vi "rs3_stream_decode3.vi"(8 "error in":errorcluster, 10 "Stream Profile Array":T2(array[cluster])=[{"ID"=1, "Profile"=389917496, "fps"=25, "RS Stream"=3, "RS Format"=0, "index"=1, "width"=1920, "height"=1080, "ppx"=0.0, "ppy"=0.0, "fx"=0.0, "fy"=0.0, "model"=0}, {"ID"=2, "Profile"=389920056, "fps"=25, "RS Stream"=3, "RS Format"=0, "index"=2, "width"=1920, "height"=1080, "ppx"=0.0, "ppy"=0.0, "fx"=0.0, "fy"=0.0, "model"=0}, {"ID"=2, "Profile"=389913400, "fps"=25, "RS Stream"=3, "RS Format"=0, "index"=2, "width"=1920, "height"=1080, "ppx"=946.5989, "ppy"=565.6723, "fx"=1415.005, "fy"=1415.005, "model"=4}, {"ID"=1, "Profile"=389905464, "fps"=25, "RS Stream"=3, "RS Format"=0, "index"=1, "width"=1920, "height"=1080, "ppx"=946.5989, "ppy"=565.6723, "fx"=1415.005, "fy"=1415.005, "model"=4}, {"ID"=1, "Profile"=389918776, "fps"=15, "RS Stream"=3, "RS Format"=0, "index"=1, "width"=1920, "height"=1080, "ppx"=0.0, "ppy"=0.0, "fx"=0.0, "fy"=0.0, "model"=0}, {"ID"=2, "Profile"=389918264, "fps"=15, "RS Stream"=3, "RS Format"=0, "index"=2, "width"=1920, "height"=1080, "ppx"=0.0, "ppy"=0.0, "fx"=0.0, "fy"=0.0, "model"=0}, {"ID"=2, "Profile"=389917240, "fps"=15, "RS Stream"=3, "RS Format"=0, "index"=2, "width"=1920, "height"=1080, "ppx"=946.5989, "ppy"=565.6723, "fx"=1415.005, "fy"=1415.005, "model"=4}, {"ID"=1, "Profile"=389916728, "fps"=15, "RS Stream"=3, "RS Format"=0, "index"=1, "width"=1920, "height"=1080, "ppx"=946.5989, "ppy"=565.6723, "fx"=1415.005, "fy"=1415.005, "model"=4}, {"ID"=1, "Profile"=389901608, "fps"=30, "RS Stream"=3, "RS Format"=0, "index"=0, "width"=1280, "height"=720, "ppx"=631.0659, "ppy"=377.11487, "fx"=943.3367, "fy"=943.3367, "model"=4}, {"ID"=1, "Profile"=389892136, "fps"=30, "RS Stream"=3, "RS Format"=0, "index"=0, "width"=1280, "height"=720, "ppx"=0.0, "ppy"=0.0, "fx"=0.0, "fy"=0.0, "model"=0}, {"ID"=1, "Profile"=389461048, "fps"=30, "RS Stream"=3, "RS Format"=0, "index"=1, "width"=1280, "height"=720, "ppx"=631.0659, "ppy"=377.11487, "fx"=943.3367, "fy"=943.3367, "model"=4}, {"ID"=2, "Profile"=389899560, "fps"=30, "RS Stream"=3, "RS Format"=0, "index"=2, "width"=1280, "height"=720, "ppx"=631.0659, "ppy"=377.11487, "fx"=943.3367, "fy"=943.3367, "model"=4}, {"ID"=1, "Profile"=389894952, "fps"=30, "RS Stream"=3, "RS Format"=0, "index"=0, "width"=1280, "height"=720, "ppx"=631.0659, "ppy"=377.11487, "fx"=943.3367, "fy"=943.3367, "model"=4}, {"ID"=1, "Profile"=389897256, "fps"=30, "RS Stream"=3, "RS Format"=0, "index"=0, "width"=1280, "height"=720, "ppx"=631.0659, "ppy"=377.11487, "fx"=943.3367, "fy"=943.3367, "model"=4}, {"ID"=1, "Profile"=389889320, "fps"=30, "RS Stream"=3, "RS Format"=0, "index"=0, "width"=1280, "height"=720, "ppx"=631.0659, "ppy"=377.11487, "fx"=943.3367, "fy"=943.3367, "model"=4}, {"ID"=1, "Profile"=389901352, "fps"=30, "RS Stream"=3, "RS Format"=0, "index"=0, "width"=1280, "height"=720, "ppx"=631.0659, "ppy"=377.11487, "fx"=943.3367, "fy"=943.3367, "model"=4}, {"ID"=1, "Profile"=389903656, "fps"=15, "RS Stream"=3, "RS Format"=0, "index"=0, "width"=1280, "height"=720, "ppx"=631.0659, "ppy"=377.11487, "fx"=943.3367, "fy"=943.3367, "model"=4}, {"ID"=1, "Profile"=389890344, "fps"=15, "RS Stream"=3, "RS Format"=0, "index"=0, "width"=1280, "height"=720, "ppx"=0.0, "ppy"=0.0, "fx"=0.0, "fy"=0.0, "model"=0}, {"ID"=1, "Profile"=389454136, "fps"=15, "RS Stream"=3, "RS Format"=0, "index"=1, "width"=1280, "height"=720, "ppx"=631.0659, "ppy"=377.11487, "fx"=943.3367, "fy"=943.3367, "model"=4}, {"ID"=2, "Profile"=389883160, "fps"=15, "RS Stream"=3, "RS Format"=0, "index"=2, "width"=1280, "height"=720, "ppx"=631.0659, "ppy"=377.11487, "fx"=943.3367, "fy"=943.3367, "model"=4}, {"ID"=1, "Profile"=389889576, "fps"=15, "RS Stream"=3, "RS Format"=0, "index"=0, "width"=1280, "height"=720, "ppx"=631.0659, "ppy"=377.11487, "fx"=943.3367, "fy"=943.3367, "model"=4}, {"ID"=1, "Profile"=389902888, "fps"=15, "RS Stream"=3, "RS Format"=0, "index"=0, "width"=1280, "height"=720, "ppx"=631.0659, "ppy"=377.11487, "fx"=943.3367, "fy"=943.3367, "model"=4}, {"ID"=1, "Profile"=389896744, "fps"=15, "RS Stream"=3, "RS Format"=0, "index"=0, "width"=1280, "height"=720, "ppx"=631.0659, "ppy"=377.11487, "fx"=943.3367, "fy"=943.3367, "model"=4}, {"ID"=1, "Profile"=389895976, "fps"=15, "RS Stream"=3, "RS Format"=0, "index"=0, "width"=1280, "height"=720, "ppx"=631.0659, "ppy"=377.11487, "fx"=943.3367, "fy"=943.3367, "model"=4}, {"ID"=1, "Profile"=389891112, "fps"=6, "RS Stream"=3, "RS Format"=0, "index"=0, "width"=1280, "height"=720, "ppx"=631.0659, "ppy"=377.11487, "fx"=943.3367, "fy"=943.3367, "model"=4}, {"ID"=1, "Profile"=389897512, "fps"=6, "RS Stream"=3, "RS Format"=0, "index"=0, "width"=1280, "height"=720, "ppx"=0.0, "ppy"=0.0, "fx"=0.0, "fy"=0.0, "model"=0}, {"ID"=1, "Profile"=389449784, "fps"=6, "RS Stream"=3, "RS Format"=0, "index"=1, "width"=1280, "height"=720, "ppx"=631.0659, "ppy"=377.11487, "fx"=943.3367, "fy"=943.3367, "model"=4}, {"ID"=2, "Profile"=389905976, "fps"=6, "RS Stream"=3, "RS Format"=0, "index"=2, "width"=1280, "height"=720, "ppx"=631.0659, "ppy"=377.11487, "fx"=943.3367, "fy"=943.3367, "model"=4}, {"ID"=1, "Profile"=389903144, "fps"=6, "RS Stream"=3, "RS Format"=0, "index"=0, "width"=1280, "height"=720, "ppx"=631.0659, "ppy"=377.11487, "fx"=943.3367, "fy"=943.3367, "model"=4}, {"ID"=1, "Profile"=389898024, "fps"=6, "RS Stream"=3, "RS Format"=0, "index"=0, "width"=1280, "height"=720, "ppx"=631.0659, "ppy"=377.11487, "fx"=943.3367, "fy"=943.3367, "model"=4}, {"ID"=1, "Profile"=389890856, "fps"=6, "RS Stream"=3, "RS Format"=0, "index"=0, "width"=1280, "height"=720, "ppx"=631.0659, "ppy"=377.11487, "fx"=943.3367, "fy"=943.3367, "model"=4}, {"ID"=1, "Profile"=389898536, "fps"=6, "RS Stream"=3, "RS Format"=0, "index"=0, "width"=1280, "height"=720, "ppx"=631.0659, "ppy"=377.11487, "fx"=943.3367, "fy"=943.3367, "model"=4}, {"ID"=1, "Profile"=389919288, "fps"=25, "RS Stream"=3, "RS Format"=0, "index"=1, "width"=960, "height"=540, "ppx"=0.0, "ppy"=0.0, "fx"=0.0, "fy"=0.0, "model"=0}, {"ID"=2, "Profile"=389919544, "fps"=25, "RS Stream"=3, "RS Format"=0, "index"=2, "width"=960, "height"=540, "ppx"=0.0, "ppy"=0.0, "fx"=0.0, "fy"=0.0, "model"=0}, {"ID"=1, "Profile"=389913656, "fps"=15, "RS Stream"=3, "RS Format"=0, "index"=1, "width"=960, "height"=540, "ppx"=0.0, "ppy"=0.0, "fx"=0.0, "fy"=0.0, "model"=0}, {"ID"=2, "Profile"=389920568, "fps"=15, "RS Stream"=3, "RS Format"=0, "index"=2, "width"=960, "height"=540, "ppx"=0.0, "ppy"=0.0, "fx"=0.0, "fy"=0.0, "model"=0}, {"ID"=1, "Profile"=389883672, "fps"=90, "RS Stream"=3, "RS Format"=0, "index"=0, "width"=848, "height"=480, "ppx"=418.04395, "ppy"=251.40993, "fx"=628.8911, "fy"=628.8911, "model"=4}, {"ID"=1, "Profile"=389883416, "fps"=90, "RS Stream"=3, "RS Format"=0, "index"=0, "width"=848, "height"=480, "ppx"=0.0, "ppy"=0.0, "fx"=0.0, "fy"=0.0, "model"=0}, {"ID"=1, "Profile"=389453112, "fps"=90, "RS Stream"=3, "RS Format"=0, "index"=1, "width"=848, "height"=480, "ppx"=418.04395, "ppy"=251.40993, "fx"=628.8911, "fy"=628.8911, "model"=4}, {"ID"=2, "Profile"=389894440, "fps"=90, "RS Stream"=3, "RS Format"=0, "index"=2, "width"=848, "height"=480, "ppx"=418.04395, "ppy"=251.40993, "fx"=628.8911, "fy"=628.8911, "model"=4}, {"ID"=1, "Profile"=389878808, "fps"=90, "RS Stream"=3, "RS Format"=0, "index"=0, "width"=848, "height"=480, "ppx"=418.04395, "ppy"=251.40993, "fx"=628.8911, "fy"=628.8911, "model"=4}, {"ID"=1, "Profile"=389887000, "fps"=90, "RS Stream"=3, "RS Format"=0, "index"=0, "width"=848, "height"=480, "ppx"=418.04395, "ppy"=251.40993, "fx"=628.8911, "fy"=628.8911, "model"=4}, {"ID"=1, "Profile"=389884952, "fps"=90, "RS Stream"=3, "RS Format"=0, "index"=0, "width"=848, "height"=480, "ppx"=418.04395, "ppy"=251.40993, "fx"=628.8911, "fy"=628.8911, "model"=4}, {"ID"=1, "Profile"=389882136, "fps"=90, "RS Stream"=3, "RS Format"=0, "index"=0, "width"=848, "height"=480, "ppx"=418.04395, "ppy"=251.40993, "fx"=628.8911, "fy"=628.8911, "model"=4}, {"ID"=1, "Profile"=389885464, "fps"=60, "RS Stream"=3, "RS Format"=0, "index"=0, "width"=848, "height"=480, "ppx"=418.04395, "ppy"=251.40993, "fx"=628.8911, "fy"=628.8911, "model"=4}, {"ID"=1, "Profile"=389885208, "fps"=60, "RS Stream"=3, "RS Format"=0, "index"=0, "width"=848, "height"=480, "ppx"=0.0, "ppy"=0.0, "fx"=0.0, "fy"=0.0, "model"=0}, {"ID"=1, "Profile"=389460536, "fps"=60, "RS Stream"=3, "RS Format"=0, "index"=1, "width"=848, "height"=480, "ppx"=418.04395, "ppy"=251.40993, "fx"=628.8911, "fy"=628.8911, "model"=4}, {"ID"=2, "Profile"=389899304, "fps"=60, "RS Stream"=3, "RS Format"=0, "index"=2, "width"=848, "height"=480, "ppx"=418.04395, "ppy"=251.40993, "fx"=628.8911, "fy"=628.8911, "model"=4}, {"ID"=1, "Profile"=389890600, "fps"=60, "RS Stream"=3, "RS Format"=0, "index"=0, "width"=848, "height"=480, "ppx"=418.04395, "ppy"=251.40993, "fx"=628.8911, "fy"=628.8911, "model"=4}, {"ID"=1, "Profile"=389886744, "fps"=60, "RS Stream"=3, "RS Format"=0, "index"=0, "width"=848, "height"=480, "ppx"=418.04395, "ppy"=251.40993, "fx"=628.8911, "fy"=628.8911, "model"=4}, {"ID"=1, "Profile"=389865480, "fps"=60, "RS Stream"=3, "RS Format"=0, "index"=0, "width"=848, "height"=480, "ppx"=418.04395, "ppy"=251.40993, "fx"=628.8911, "fy"=628.8911, "model"=4}, {"ID"=1, "Profile"=389883928, "fps"=60, "RS Stream"=3, "RS Format"=0, "index"=0, "width"=848, "height"=480, "ppx"=418.04395, "ppy"=251.40993, "fx"=628.8911, "fy"=628.8911, "model"=4}, {"ID"=1, "Profile"=389900072, "fps"=30, "RS Stream"=3, "RS Format"=0, "index"=0, "width"=848, "height"=480, "ppx"=418.04395, "ppy"=251.40993, "fx"=628.8911, "fy"=628.8911, "model"=4}, {"ID"=1, "Profile"=389891880, "fps"=30, "RS Stream"=3, "RS Format"=0, "index"=0, "width"=848, "height"=480, "ppx"=0.0, "ppy"=0.0, "fx"=0.0, "fy"=0.0, "model"=0}, {"ID"=1, "Profile"=389453880, "fps"=30, "RS Stream"=3, "RS Format"=0, "index"=1, "width"=848, "height"=480, "ppx"=418.04395, "ppy"=251.40993, "fx"=628.8911, "fy"=628.8911, "model"=4}, {"ID"=2, "Profile"=389896232, "fps"=30, "RS Stream"=3, "RS Format"=0, "index"=2, "width"=848, "height"=480, "ppx"=418.04395, "ppy"=251.40993, "fx"=628.8911, "fy"=628.8911, "model"=4}, {"ID"=1, "Profile"=389904680, "fps"=30, "RS Stream"=3, "RS Format"=0, "index"=0, "width"=848, "height"=480, "ppx"=418.04395, "ppy"=251.40993, "fx"=628.8911, "fy"=628.8911, "model"=4}, {"ID"=1, "Profile"=389900584, "fps"=30, "RS Stream"=3, "RS Format"=0, "index"=0, "width"=848, "height"=480, "ppx"=418.04395, "ppy"=251.40993, "fx"=628.8911, "fy"=628.8911, "model"=4}, {"ID"=1, "Profile"=389897768, "fps"=30, "RS Stream"=3, "RS Format"=0, "index"=0, "width"=848, "height"=480, "ppx"=418.04395, "ppy"=251.40993, "fx"=628.8911, "fy"=628.8911, "model"=4}, {"ID"=1, "Profile"=389902120, "fps"=30, "RS Stream"=3, "RS Format"=0, "index"=0, "width"=848, "height"=480, "ppx"=418.04395, "ppy"=251.40993, "fx"=628.8911, "fy"=628.8911, "model"=4}, {"ID"=1, "Profile"=389900840, "fps"=15, "RS Stream"=3, "RS Format"=0, "index"=0, "width"=848, "height"=480, "ppx"=418.04395, "ppy"=251.40993, "fx"=628.8911, "fy"=628.8911, "model"=4}, {"ID"=1, "Profile"=389897000, "fps"=15, "RS Stream"=3, "RS Format"=0, "index"=0, "width"=848, "height"=480, "ppx"=0.0, "ppy"=0.0, "fx"=0.0, "fy"=0.0, "model"=0}, {"ID"=2, "Profile"=389896488, "fps"=15, "RS Stream"=3, "RS Format"=0, "index"=2, "width"=848, "height"=480, "ppx"=418.04395, "ppy"=251.40993, "fx"=628.8911, "fy"=628.8911, "model"=4}, {"ID"=1, "Profile"=389449528, "fps"=15, "RS Stream"=3, "RS Format"=0, "index"=1, "width"=848, "height"=480, "ppx"=418.04395, "ppy"=251.40993, "fx"=628.8911, "fy"=628.8911, "model"=4}, {"ID"=1, "Profile"=389902376, "fps"=15, "RS Stream"=3, "RS Format"=0, "index"=0, "width"=848, "height"=480, "ppx"=418.04395, "ppy"=251.40993, "fx"=628.8911, "fy"=628.8911, "model"=4}, {"ID"=1, "Profile"=389903400, "fps"=15, "RS Stream"=3, "RS Format"=0, "index"=0, "width"=848, "height"=480, "ppx"=418.04395, "ppy"=251.40993, "fx"=628.8911, "fy"=628.8911, "model"=4}, {"ID"=1, "Profile"=389893928, "fps"=15, "RS Stream"=3, "RS Format"=0, "index"=0, "width"=848, "height"=480, "ppx"=418.04395, "ppy"=251.40993, "fx"=628.8911, "fy"=628.8911, "model"=4}, {"ID"=1, "Profile"=389903912, "fps"=15, "RS Stream"=3, "RS Format"=0, "index"=0, "width"=848, "height"=480, "ppx"=418.04395, "ppy"=251.40993, "fx"=628.8911, "fy"=628.8911, "model"=4}, {"ID"=1, "Profile"=389901096, "fps"=6, "RS Stream"=3, "RS Format"=0, "index"=0, "width"=848, "height"=480, "ppx"=418.04395, "ppy"=251.40993, "fx"=628.8911, "fy"=628.8911, "model"=4}, {"ID"=1, "Profile"=389895720, "fps"=6, "RS Stream"=3, "RS Format"=0, "index"=0, "width"=848, "height"=480, "ppx"=0.0, "ppy"=0.0, "fx"=0.0, "fy"=0.0, "model"=0}, {"ID"=1, "Profile"=389445688, "fps"=6, "RS Stream"=3, "RS Format"=0, "index"=1, "width"=848, "height"=480, "ppx"=418.04395, "ppy"=251.40993, "fx"=628.8911, "fy"=628.8911, "model"=4}, {"ID"=2, "Profile"=389898280, "fps"=6, "RS Stream"=3, "RS Format"=0, "index"=2, "width"=848, "height"=480, "ppx"=418.04395, "ppy"=251.40993, "fx"=628.8911, "fy"=628.8911, "model"=4}, {"ID"=1, "Profile"=389902632, "fps"=6, "RS Stream"=3, "RS Format"=0, "index"=0, "width"=848, "height"=480, "ppx"=418.04395, "ppy"=251.40993, "fx"=628.8911, "fy"=628.8911, "model"=4}, {"ID"=1, "Profile"=389892392, "fps"=6, "RS Stream"=3, "RS Format"=0, "index"=0, "width"=848, "height"=480, "ppx"=418.04395, "ppy"=251.40993, "fx"=628.8911, "fy"=628.8911, "model"=4}, {"ID"=1, "Profile"=389901864, "fps"=6, "RS Stream"=3, "RS Format"=0, "index"=0, "width"=848, "height"=480, "ppx"=418.04395, "ppy"=251.40993, "fx"=628.8911, "fy"=628.8911, "model"=4}, {"ID"=1, "Profile"=389899816, "fps"=6, "RS Stream"=3, "RS Format"=0, "index"=0, "width"=848, "height"=480, "ppx"=418.04395, "ppy"=251.40993, "fx"=628.8911, "fy"=628.8911, "model"=4}, {"ID"=1, "Profile"=389874200, "fps"=90, "RS Stream"=3, "RS Format"=0, "index"=0, "width"=640, "height"=480, "ppx"=314.04395, "ppy"=251.40993, "fx"=628.8911, "fy"=628.8911, "model"=4}, {"ID"=1, "Profile"=389880600, "fps"=90, "RS Stream"=3, "RS Format"=0, "index"=0, "width"=640, "height"=480, "ppx"=0.0, "ppy"=0.0, "fx"=0.0, "fy"=0.0, "model"=0}, {"ID"=1, "Profile"=389458744, "fps"=90, "RS Stream"=3, "RS Format"=0, "index"=1, "width"=640, "height"=480, "ppx"=314.04395, "ppy"=251.40993, "fx"=628.8911, "fy"=628.8911, "model"=4}, {"ID"=2, "Profile"=389893160, "fps"=90, "RS Stream"=3, "RS Format"=0, "index"=2, "width"=640, "height"=480, "ppx"=314.04395, "ppy"=251.40993, "fx"=628.8911, "fy"=628.8911, "model"=4}, {"ID"=1, "Profile"=389882904, "fps"=90, "RS Stream"=3, "RS Format"=0, "index"=0, "width"=640, "height"=480, "ppx"=314.04395, "ppy"=251.40993, "fx"=628.8911, "fy"=628.8911, "model"=4}, {"ID"=1, "Profile"=389880856, "fps"=90, "RS Stream"=3, "RS Format"=0, "index"=0, "width"=640, "height"=480, "ppx"=314.04395, "ppy"=251.40993, "fx"=628.8911, "fy"=628.8911, "model"=4}, {"ID"=1, "Profile"=389875224, "fps"=90, "RS Stream"=3, "RS Format"=0, "index"=0, "width"=640, "height"=480, "ppx"=314.04395, "ppy"=251.40993, "fx"=628.8911, "fy"=628.8911, "model"=4}, {"ID"=1, "Profile"=389875992, "fps"=90, "RS Stream"=3, "RS Format"=0, "index"=0, "width"=640, "height"=480, "ppx"=314.04395, "ppy"=251.40993, "fx"=628.8911, "fy"=628.8911, "model"=4}, {"ID"=1, "Profile"=389876760, "fps"=60, "RS Stream"=3, "RS Format"=0, "index"=0, "width"=640, "height"=480, "ppx"=314.04395, "ppy"=251.40993, "fx"=628.8911, "fy"=628.8911, "model"=4}, {"ID"=1, "Profile"=389881880, "fps"=60, "RS Stream"=3, "RS Format"=0, "index"=0, "width"=640, "height"=480, "ppx"=0.0, "ppy"=0.0, "fx"=0.0, "fy"=0.0, "model"=0}, {"ID"=2, "Profile"=389895208, "fps"=60, "RS Stream"=3, "RS Format"=0, "index"=2, "width"=640, "height"=480, "ppx"=314.04395, "ppy"=251.40993, "fx"=628.8911, "fy"=628.8911, "model"=4}, {"ID"=1, "Profile"=389446968, "fps"=60, "RS Stream"=3, "RS Format"=0, "index"=1, "width"=640, "height"=480, "ppx"=314.04395, "ppy"=251.40993, "fx"=628.8911, "fy"=628.8911, "model"=4}, {"ID"=1, "Profile"=389885976, "fps"=60, "RS Stream"=3, "RS Format"=0, "index"=0, "width"=640, "height"=480, "ppx"=314.04395, "ppy"=251.40993, "fx"=628.8911, "fy"=628.8911, "model"=4}, {"ID"=1, "Profile"=389874456, "fps"=60, "RS Stream"=3, "RS Format"=0, "index"=0, "width"=640, "height"=480, "ppx"=314.04395, "ppy"=251.40993, "fx"=628.8911, "fy"=628.8911, "model"=4}, {"ID"=1, "Profile"=389874968, "fps"=60, "RS Stream"=3, "RS Format"=0, "index"=0, "width"=640, "height"=480, "ppx"=314.04395, "ppy"=251.40993, "fx"=628.8911, "fy"=628.8911, "model"=4}, {"ID"=1, "Profile"=389878296, "fps"=60, "RS Stream"=3, "RS Format"=0, "index"=0, "width"=640, "height"=480, "ppx"=314.04395, "ppy"=251.40993, "fx"=628.8911, "fy"=628.8911, "model"=4}, {"ID"=1, "Profile"=389872920, "fps"=30, "RS Stream"=3, "RS Format"=0, "index"=0, "width"=640, "height"=480, "ppx"=314.04395, "ppy"=251.40993, "fx"=628.8911, "fy"=628.8911, "model"=4}, {"ID"=1, "Profile"=389872664, "fps"=30, "RS Stream"=3, "RS Format"=0, "index"=0, "width"=640, "height"=480, "ppx"=0.0, "ppy"=0.0, "fx"=0.0, "fy"=0.0, "model"=0}, {"ID"=2, "Profile"=389893672, "fps"=30, "RS Stream"=3, "RS Format"=0, "index"=2, "width"=640, "height"=480, "ppx"=314.04395, "ppy"=251.40993, "fx"=628.8911, "fy"=628.8911, "model"=4}, {"ID"=1, "Profile"=389459000, "fps"=30, "RS Stream"=3, "RS Format"=0, "index"=1, "width"=640, "height"=480, "ppx"=314.04395, "ppy"=251.40993, "fx"=628.8911, "fy"=628.8911, "model"=4}, {"ID"=1, "Profile"=389877784, "fps"=30, "RS Stream"=3, "RS Format"=0, "index"=0, "width"=640, "height"=480, "ppx"=314.04395, "ppy"=251.40993, "fx"=628.8911, "fy"=628.8911, "model"=4}, {"ID"=1, "Profile"=389888024, "fps"=30, "RS Stream"=3, "RS Format"=0, "index"=0, "width"=640, "height"=480, "ppx"=314.04395, "ppy"=251.40993, "fx"=628.8911, "fy"=628.8911, "model"=4}, {"ID"=1, "Profile"=389888536, "fps"=30, "RS Stream"=3, "RS Format"=0, "index"=0, "width"=640, "height"=480, "ppx"=314.04395, "ppy"=251.40993, "fx"=628.8911, "fy"=628.8911, "model"=4}, {"ID"=1, "Profile"=389877016, "fps"=30, "RS Stream"=3, "RS Format"=0, "index"=0, "width"=640, "height"=480, "ppx"=314.04395, "ppy"=251.40993, "fx"=628.8911, "fy"=628.8911, "model"=4}, {"ID"=1, "Profile"=389884184, "fps"=15, "RS Stream"=3, "RS Format"=0, "index"=0, "width"=640, "height"=480, "ppx"=314.04395, "ppy"=251.40993, "fx"=628.8911, "fy"=628.8911, "model"=4}, {"ID"=1, "Profile"=389878552, "fps"=15, "RS Stream"=3, "RS Format"=0, "index"=0, "width"=640, "height"=480, "ppx"=0.0, "ppy"=0.0, "fx"=0.0, "fy"=0.0, "model"=0}, {"ID"=2, "Profile"=389899048, "fps"=15, "RS Stream"=3, "RS Format"=0, "index"=2, "width"=640, "height"=480, "ppx"=314.04395, "ppy"=251.40993, "fx"=628.8911, "fy"=628.8911, "model"=4}, {"ID"=1, "Profile"=389459256, "fps"=15, "RS Stream"=3, "RS Format"=0, "index"=1, "width"=640, "height"=480, "ppx"=314.04395, "ppy"=251.40993, "fx"=628.8911, "fy"=628.8911, "model"=4}, {"ID"=1, "Profile"=389878040, "fps"=15, "RS Stream"=3, "RS Format"=0, "index"=0, "width"=640, "height"=480, "ppx"=314.04395, "ppy"=251.40993, "fx"=628.8911, "fy"=628.8911, "model"=4}, {"ID"=1, "Profile"=389886488, "fps"=15, "RS Stream"=3, "RS Format"=0, "index"=0, "width"=640, "height"=480, "ppx"=314.04395, "ppy"=251.40993, "fx"=628.8911, "fy"=628.8911, "model"=4}, {"ID"=1, "Profile"=389877528, "fps"=15, "RS Stream"=3, "RS Format"=0, "index"=0, "width"=640, "height"=480, "ppx"=314.04395, "ppy"=251.40993, "fx"=628.8911, "fy"=628.8911, "model"=4}, {"ID"=1, "Profile"=389886232, "fps"=15, "RS Stream"=3, "RS Format"=0, "index"=0, "width"=640, "height"=480, "ppx"=314.04395, "ppy"=251.40993, "fx"=628.8911, "fy"=628.8911, "model"=4}, {"ID"=1, "Profile"=389884696, "fps"=6, "RS Stream"=3, "RS Format"=0, "index"=0, "width"=640, "height"=480, "ppx"=314.04395, "ppy"=251.40993, "fx"=628.8911, "fy"=628.8911, "model"=4}, {"ID"=1, "Profile"=389882392, "fps"=6, "RS Stream"=3, "RS Format"=0, "index"=0, "width"=640, "height"=480, "ppx"=0.0, "ppy"=0.0, "fx"=0.0, "fy"=0.0, "model"=0}, {"ID"=2, "Profile"=389894184, "fps"=6, "RS Stream"=3, "RS Format"=0, "index"=2, "width"=640, "height"=480, "ppx"=314.04395, "ppy"=251.40993, "fx"=628.8911, "fy"=628.8911, "model"=4}, {"ID"=1, "Profile"=389460280, "fps"=6, "RS Stream"=3, "RS Format"=0, "index"=1, "width"=640, "height"=480, "ppx"=314.04395, "ppy"=251.40993, "fx"=628.8911, "fy"=628.8911, "model"=4}, {"ID"=1, "Profile"=389880344, "fps"=6, "RS Stream"=3, "RS Format"=0, "index"=0, "width"=640, "height"=480, "ppx"=314.04395, "ppy"=251.40993, "fx"=628.8911, "fy"=628.8911, "model"=4}, {"ID"=1, "Profile"=389879832, "fps"=6, "RS Stream"=3, "RS Format"=0, "index"=0, "width"=640, "height"=480, "ppx"=314.04395, "ppy"=251.40993, "fx"=628.8911, "fy"=628.8911, "model"=4}, {"ID"=1, "Profile"=389884440, "fps"=6, "RS Stream"=3, "RS Format"=0, "index"=0, "width"=640, "height"=480, "ppx"=314.04395, "ppy"=251.40993, "fx"=628.8911, "fy"=628.8911, "model"=4}, {"ID"=1, "Profile"=389876248, "fps"=6, "RS Stream"=3, "RS Format"=0, "index"=0, "width"=640, "height"=480, "ppx"=314.04395, "ppy"=251.40993, "fx"=628.8911, "fy"=628.8911, "model"=4}, {"ID"=1, "Profile"=389863944, "fps"=90, "RS Stream"=3, "RS Format"=0, "index"=0, "width"=640, "height"=360, "ppx"=315.53296, "ppy"=188.55743, "fx"=471.66833, "fy"=471.66833, "model"=4}, {"ID"=1, "Profile"=389863688, "fps"=90, "RS Stream"=3, "RS Format"=0, "index"=0, "width"=640, "height"=360, "ppx"=0.0, "ppy"=0.0, "fx"=0.0, "fy"=0.0, "model"=0}, {"ID"=2, "Profile"=389889064, "fps"=90, "RS Stream"=3, "RS Format"=0, "index"=2, "width"=640, "height"=360, "ppx"=315.53296, "ppy"=188.55743, "fx"=471.66833, "fy"=471.66833, "model"=4}, {"ID"=1, "Profile"=389461304, "fps"=90, "RS Stream"=3, "RS Format"=0, "index"=1, "width"=640, "height"=360, "ppx"=315.53296, "ppy"=188.55743, "fx"=471.66833, "fy"=471.66833, "model"=4}, {"ID"=1, "Profile"=389866760, "fps"=90, "RS Stream"=3, "RS Format"=0, "index"=0, "width"=640, "height"=360, "ppx"=315.53296, "ppy"=188.55743, "fx"=471.66833, "fy"=471.66833, "model"=4}, {"ID"=1, "Profile"=389864456, "fps"=90, "RS Stream"=3, "RS Format"=0, "index"=0, "width"=640, "height"=360, "ppx"=315.53296, "ppy"=188.55743, "fx"=471.66833, "fy"=471.66833, "model"=4}, {"ID"=1, "Profile"=389867528, "fps"=90, "RS Stream"=3, "RS Format"=0, "index"=0, "width"=640, "height"=360, "ppx"=315.53296, "ppy"=188.55743, "fx"=471.66833, "fy"=471.66833, "model"=4}, {"ID"=1, "Profile"=389863432, "fps"=90, "RS Stream"=3, "RS Format"=0, "index"=0, "width"=640, "height"=360, "ppx"=315.53296, "ppy"=188.55743, "fx"=471.66833, "fy"=471.66833, "model"=4}, {"ID"=1, "Profile"=389887512, "fps"=60, "RS Stream"=3, "RS Format"=0, "index"=0, "width"=640, "height"=360, "ppx"=315.53296, "ppy"=188.55743, "fx"=471.66833, "fy"=471.66833, "model"=4}, {"ID"=1, "Profile"=389451576, "fps"=60, "RS Stream"=3, "RS Format"=0, "index"=0, "width"=640, "height"=360, "ppx"=0.0, "ppy"=0.0, "fx"=0.0, "fy"=0.0, "model"=0}, {"ID"=1, "Profile"=389446712, "fps"=60, "RS Stream"=3, "RS Format"=0, "index"=1, "width"=640, "height"=360, "ppx"=315.53296, "ppy"=188.55743, "fx"=471.66833, "fy"=471.66833, "model"=4}, {"ID"=2, "Profile"=389891368, "fps"=60, "RS Stream"=3, "RS Format"=0, "index"=2, "width"=640, "height"=360, "ppx"=315.53296, "ppy"=188.55743, "fx"=471.66833, "fy"=471.66833, "model"=4}, {"ID"=1, "Profile"=389873176, "fps"=60, "RS Stream"=3, "RS Format"=0, "index"=0, "width"=640, "height"=360, "ppx"=315.53296, "ppy"=188.55743, "fx"=471.66833, "fy"=471.66833, "model"=4}, {"ID"=1, "Profile"=389882648, "fps"=60, "RS Stream"=3, "RS Format"=0, "index"=0, "width"=640, "height"=360, "ppx"=315.53296, "ppy"=188.55743, "fx"=471.66833, "fy"=471.66833, "model"=4}, {"ID"=1, "Profile"=389879576, "fps"=60, "RS Stream"=3, "RS Format"=0, "index"=0, "width"=640, "height"=360, "ppx"=315.53296, "ppy"=188.55743, "fx"=471.66833, "fy"=471.66833, "model"=4}, {"ID"=1, "Profile"=389863176, "fps"=60, "RS Stream"=3, "RS Format"=0, "index"=0, "width"=640, "height"=360, "ppx"=315.53296, "ppy"=188.55743, "fx"=471.66833, "fy"=471.66833, "model"=4}, {"ID"=1, "Profile"=389873432, "fps"=30, "RS Stream"=3, "RS Format"=0, "index"=0, "width"=640, "height"=360, "ppx"=315.53296, "ppy"=188.55743, "fx"=471.66833, "fy"=471.66833, "model"=4}, {"ID"=1, "Profile"=389888280, "fps"=30, "RS Stream"=3, "RS Format"=0, "index"=0, "width"=640, "height"=360, "ppx"=0.0, "ppy"=0.0, "fx"=0.0, "fy"=0.0, "model"=0}, {"ID"=2, "Profile"=389904936, "fps"=30, "RS Stream"=3, "RS Format"=0, "index"=2, "width"=640, "height"=360, "ppx"=315.53296, "ppy"=188.55743, "fx"=471.66833, "fy"=471.66833, "model"=4}, {"ID"=1, "Profile"=389456184, "fps"=30, "RS Stream"=3, "RS Format"=0, "index"=1, "width"=640, "height"=360, "ppx"=315.53296, "ppy"=188.55743, "fx"=471.66833, "fy"=471.66833, "model"=4}, {"ID"=1, "Profile"=389879064, "fps"=30, "RS Stream"=3, "RS Format"=0, "index"=0, "width"=640, "height"=360, "ppx"=315.53296, "ppy"=188.55743, "fx"=471.66833, "fy"=471.66833, "model"=4}, {"ID"=1, "Profile"=389881624, "fps"=30, "RS Stream"=3, "RS Format"=0, "index"=0, "width"=640, "height"=360, "ppx"=315.53296, "ppy"=188.55743, "fx"=471.66833, "fy"=471.66833, "model"=4}, {"ID"=1, "Profile"=389875480, "fps"=30, "RS Stream"=3, "RS Format"=0, "index"=0, "width"=640, "height"=360, "ppx"=315.53296, "ppy"=188.55743, "fx"=471.66833, "fy"=471.66833, "model"=4}, {"ID"=1, "Profile"=389881368, "fps"=30, "RS Stream"=3, "RS Format"=0, "index"=0, "width"=640, "height"=360, "ppx"=315.53296, "ppy"=188.55743, "fx"=471.66833, "fy"=471.66833, "model"=4}, {"ID"=1, "Profile"=389885720, "fps"=15, "RS Stream"=3, "RS Format"=0, "index"=0, "width"=640, "height"=360, "ppx"=315.53296, "ppy"=188.55743, "fx"=471.66833, "fy"=471.66833, "model"=4}, {"ID"=1, "Profile"=389875736, "fps"=15, "RS Stream"=3, "RS Format"=0, "index"=0, "width"=640, "height"=360, "ppx"=0.0, "ppy"=0.0, "fx"=0.0, "fy"=0.0, "model"=0}, {"ID"=1, "Profile"=389459512, "fps"=15, "RS Stream"=3, "RS Format"=0, "index"=1, "width"=640, "height"=360, "ppx"=315.53296, "ppy"=188.55743, "fx"=471.66833, "fy"=471.66833, "model"=4}, {"ID"=2, "Profile"=389892904, "fps"=15, "RS Stream"=3, "RS Format"=0, "index"=2, "width"=640, "height"=360, "ppx"=315.53296, "ppy"=188.55743, "fx"=471.66833, "fy"=471.66833, "model"=4}, {"ID"=1, "Profile"=389881112, "fps"=15, "RS Stream"=3, "RS Format"=0, "index"=0, "width"=640, "height"=360, "ppx"=315.53296, "ppy"=188.55743, "fx"=471.66833, "fy"=471.66833, "model"=4}, {"ID"=1, "Profile"=389876504, "fps"=15, "RS Stream"=3, "RS Format"=0, "index"=0, "width"=640, "height"=360, "ppx"=315.53296, "ppy"=188.55743, "fx"=471.66833, "fy"=471.66833, "model"=4}, {"ID"=1, "Profile"=389880088, "fps"=15, "RS Stream"=3, "RS Format"=0, "index"=0, "width"=640, "height"=360, "ppx"=315.53296, "ppy"=188.55743, "fx"=471.66833, "fy"=471.66833, "model"=4}, {"ID"=1, "Profile"=389879320, "fps"=15, "RS Stream"=3, "RS Format"=0, "index"=0, "width"=640, "height"=360, "ppx"=315.53296, "ppy"=188.55743, "fx"=471.66833, "fy"=471.66833, "model"=4}, {"ID"=1, "Profile"=389877272, "fps"=6, "RS Stream"=3, "RS Format"=0, "index"=0, "width"=640, "height"=360, "ppx"=315.53296, "ppy"=188.55743, "fx"=471.66833, "fy"=471.66833, "model"=4}, {"ID"=1, "Profile"=389887768, "fps"=6, "RS Stream"=3, "RS Format"=0, "index"=0, "width"=640, "height"=360, "ppx"=0.0, "ppy"=0.0, "fx"=0.0, "fy"=0.0, "model"=0}, {"ID"=1, "Profile"=389456440, "fps"=6, "RS Stream"=3, "RS Format"=0, "index"=1, "width"=640, "height"=360, "ppx"=315.53296, "ppy"=188.55743, "fx"=471.66833, "fy"=471.66833, "model"=4}, {"ID"=2, "Profile"=389893416, "fps"=6, "RS Stream"=3, "RS Format"=0, "index"=2, "width"=640, "height"=360, "ppx"=315.53296, "ppy"=188.55743, "fx"=471.66833, "fy"=471.66833, "model"=4}, {"ID"=1, "Profile"=389874712, "fps"=6, "RS Stream"=3, "RS Format"=0, "index"=0, "width"=640, "height"=360, "ppx"=315.53296, "ppy"=188.55743, "fx"=471.66833, "fy"=471.66833, "model"=4}, {"ID"=1, "Profile"=389887256, "fps"=6, "RS Stream"=3, "RS Format"=0, "index"=0, "width"=640, "height"=360, "ppx"=315.53296, "ppy"=188.55743, "fx"=471.66833, "fy"=471.66833, "model"=4}, {"ID"=1, "Profile"=389873944, "fps"=6, "RS Stream"=3, "RS Format"=0, "index"=0, "width"=640, "height"=360, "ppx"=315.53296, "ppy"=188.55743, "fx"=471.66833, "fy"=471.66833, "model"=4}, {"ID"=1, "Profile"=389873688, "fps"=6, "RS Stream"=3, "RS Format"=0, "index"=0, "width"=640, "height"=360, "ppx"=315.53296, "ppy"=188.55743, "fx"=471.66833, "fy"=471.66833, "model"=4}, {"ID"=1, "Profile"=389864200, "fps"=90, "RS Stream"=3, "RS Format"=0, "index"=0, "width"=480, "height"=270, "ppx"=236.64972, "ppy"=141.41808, "fx"=353.75125, "fy"=353.75125, "model"=4}, {"ID"=1, "Profile"=389860872, "fps"=90, "RS Stream"=3, "RS Format"=0, "index"=0, "width"=480, "height"=270, "ppx"=0.0, "ppy"=0.0, "fx"=0.0, "fy"=0.0, "model"=0}, {"ID"=2, "Profile"=389891624, "fps"=90, "RS Stream"=3, "RS Format"=0, "index"=2, "width"=480, "height"=270, "ppx"=236.64972, "ppy"=141.41808, "fx"=353.75125, "fy"=353.75125, "model"=4}, {"ID"=1, "Profile"=389455928, "fps"=90, "RS Stream"=3, "RS Format"=0, "index"=1, "width"=480, "height"=270, "ppx"=236.64972, "ppy"=141.41808, "fx"=353.75125, "fy"=353.75125, "model"=4}, {"ID"=1, "Profile"=389858056, "fps"=90, "RS Stream"=3, "RS Format"=0, "index"=0, "width"=480, "height"=270, "ppx"=236.64972, "ppy"=141.41808, "fx"=353.75125, "fy"=353.75125, "model"=4}, {"ID"=1, "Profile"=389857800, "fps"=90, "RS Stream"=3, "RS Format"=0, "index"=0, "width"=480, "height"=270, "ppx"=236.64972, "ppy"=141.41808, "fx"=353.75125, "fy"=353.75125, "model"=4}, {"ID"=1, "Profile"=389857544, "fps"=90, "RS Stream"=3, "RS Format"=0, "index"=0, "width"=480, "height"=270, "ppx"=236.64972, "ppy"=141.41808, "fx"=353.75125, "fy"=353.75125, "model"=4}, {"ID"=1, "Profile"=389861896, "fps"=90, "RS Stream"=3, "RS Format"=0, "index"=0, "width"=480, "height"=270, "ppx"=236.64972, "ppy"=141.41808, "fx"=353.75125, "fy"=353.75125, "model"=4}, {"ID"=1, "Profile"=389856776, "fps"=60, "RS Stream"=3, "RS Format"=0, "index"=0, "width"=480, "height"=270, "ppx"=236.64972, "ppy"=141.41808, "fx"=353.75125, "fy"=353.75125, "model"=4}, {"ID"=1, "Profile"=389870344, "fps"=60, "RS Stream"=3, "RS Format"=0, "index"=0, "width"=480, "height"=270, "ppx"=0.0, "ppy"=0.0, "fx"=0.0, "fy"=0.0, "model"=0}, {"ID"=2, "Profile"=389900328, "fps"=60, "RS Stream"=3, "RS Format"=0, "index"=2, "width"=480, "height"=270, "ppx"=236.64972, "ppy"=141.41808, "fx"=353.75125, "fy"=353.75125, "model"=4}, {"ID"=1, "Profile"=389457208, "fps"=60, "RS Stream"=3, "RS Format"=0, "index"=1, "width"=480, "height"=270, "ppx"=236.64972, "ppy"=141.41808, "fx"=353.75125, "fy"=353.75125, "model"=4}, {"ID"=1, "Profile"=389870600, "fps"=60, "RS Stream"=3, "RS Format"=0, "index"=0, "width"=480, "height"=270, "ppx"=236.64972, "ppy"=141.41808, "fx"=353.75125, "fy"=353.75125, "model"=4}, {"ID"=1, "Profile"=389865992, "fps"=60, "RS Stream"=3, "RS Format"=0, "index"=0, "width"=480, "height"=270, "ppx"=236.64972, "ppy"=141.41808, "fx"=353.75125, "fy"=353.75125, "model"=4}, {"ID"=1, "Profile"=389859336, "fps"=60, "RS Stream"=3, "RS Format"=0, "index"=0, "width"=480, "height"=270, "ppx"=236.64972, "ppy"=141.41808, "fx"=353.75125, "fy"=353.75125, "model"=4}, {"ID"=1, "Profile"=389867784, "fps"=60, "RS Stream"=3, "RS Format"=0, "index"=0, "width"=480, "height"=270, "ppx"=236.64972, "ppy"=141.41808, "fx"=353.75125, "fy"=353.75125, "model"=4}, {"ID"=1, "Profile"=389872136, "fps"=30, "RS Stream"=3, "RS Format"=0, "index"=0, "width"=480, "height"=270, "ppx"=236.64972, "ppy"=141.41808, "fx"=353.75125, "fy"=353.75125, "model"=4}, {"ID"=1, "Profile"=389861128, "fps"=30, "RS Stream"=3, "RS Format"=0, "index"=0, "width"=480, "height"=270, "ppx"=0.0, "ppy"=0.0, "fx"=0.0, "fy"=0.0, "model"=0}, {"ID"=2, "Profile"=389889832, "fps"=30, "RS Stream"=3, "RS Format"=0, "index"=2, "width"=480, "height"=270, "ppx"=236.64972, "ppy"=141.41808, "fx"=353.75125, "fy"=353.75125, "model"=4}, {"ID"=1, "Profile"=389450808, "fps"=30, "RS Stream"=3, "RS Format"=0, "index"=1, "width"=480, "height"=270, "ppx"=236.64972, "ppy"=141.41808, "fx"=353.75125, "fy"=353.75125, "model"=4}, {"ID"=1, "Profile"=389856264, "fps"=30, "RS Stream"=3, "RS Format"=0, "index"=0, "width"=480, "height"=270, "ppx"=236.64972, "ppy"=141.41808, "fx"=353.75125, "fy"=353.75125, "model"=4}, {"ID"=1, "Profile"=389865224, "fps"=30, "RS Stream"=3, "RS Format"=0, "index"=0, "width"=480, "height"=270, "ppx"=236.64972, "ppy"=141.41808, "fx"=353.75125, "fy"=353.75125, "model"=4}, {"ID"=1, "Profile"=389870856, "fps"=30, "RS Stream"=3, "RS Format"=0, "index"=0, "width"=480, "height"=270, "ppx"=236.64972, "ppy"=141.41808, "fx"=353.75125, "fy"=353.75125, "model"=4}, {"ID"=1, "Profile"=389860616, "fps"=30, "RS Stream"=3, "RS Format"=0, "index"=0, "width"=480, "height"=270, "ppx"=236.64972, "ppy"=141.41808, "fx"=353.75125, "fy"=353.75125, "model"=4}, {"ID"=1, "Profile"=389868040, "fps"=15, "RS Stream"=3, "RS Format"=0, "index"=0, "width"=480, "height"=270, "ppx"=236.64972, "ppy"=141.41808, "fx"=353.75125, "fy"=353.75125, "model"=4}, {"ID"=1, "Profile"=389857032, "fps"=15, "RS Stream"=3, "RS Format"=0, "index"=0, "width"=480, "height"=270, "ppx"=0.0, "ppy"=0.0, "fx"=0.0, "fy"=0.0, "model"=0}, {"ID"=1, "Profile"=389449016, "fps"=15, "RS Stream"=3, "RS Format"=0, "index"=1, "width"=480, "height"=270, "ppx"=236.64972, "ppy"=141.41808, "fx"=353.75125, "fy"=353.75125, "model"=4}, {"ID"=2, "Profile"=389894696, "fps"=15, "RS Stream"=3, "RS Format"=0, "index"=2, "width"=480, "height"=270, "ppx"=236.64972, "ppy"=141.41808, "fx"=353.75125, "fy"=353.75125, "model"=4}, {"ID"=1, "Profile"=389859592, "fps"=15, "RS Stream"=3, "RS Format"=0, "index"=0, "width"=480, "height"=270, "ppx"=236.64972, "ppy"=141.41808, "fx"=353.75125, "fy"=353.75125, "model"=4}, {"ID"=1, "Profile"=389871112, "fps"=15, "RS Stream"=3, "RS Format"=0, "index"=0, "width"=480, "height"=270, "ppx"=236.64972, "ppy"=141.41808, "fx"=353.75125, "fy"=353.75125, "model"=4}, {"ID"=1, "Profile"=389858312, "fps"=15, "RS Stream"=3, "RS Format"=0, "index"=0, "width"=480, "height"=270, "ppx"=236.64972, "ppy"=141.41808, "fx"=353.75125, "fy"=353.75125, "model"=4}, {"ID"=1, "Profile"=389862664, "fps"=15, "RS Stream"=3, "RS Format"=0, "index"=0, "width"=480, "height"=270, "ppx"=236.64972, "ppy"=141.41808, "fx"=353.75125, "fy"=353.75125, "model"=4}, {"ID"=1, "Profile"=389860360, "fps"=6, "RS Stream"=3, "RS Format"=0, "index"=0, "width"=480, "height"=270, "ppx"=236.64972, "ppy"=141.41808, "fx"=353.75125, "fy"=353.75125, "model"=4}, {"ID"=1, "Profile"=389862920, "fps"=6, "RS Stream"=3, "RS Format"=0, "index"=0, "width"=480, "height"=270, "ppx"=0.0, "ppy"=0.0, "fx"=0.0, "fy"=0.0, "model"=0}, {"ID"=1, "Profile"=389458488, "fps"=6, "RS Stream"=3, "RS Format"=0, "index"=1, "width"=480, "height"=270, "ppx"=236.64972, "ppy"=141.41808, "fx"=353.75125, "fy"=353.75125, "model"=4}, {"ID"=2, "Profile"=389890088, "fps"=6, "RS Stream"=3, "RS Format"=0, "index"=2, "width"=480, "height"=270, "ppx"=236.64972, "ppy"=141.41808, "fx"=353.75125, "fy"=353.75125, "model"=4}, {"ID"=1, "Profile"=389860104, "fps"=6, "RS Stream"=3, "RS Format"=0, "index"=0, "width"=480, "height"=270, "ppx"=236.64972, "ppy"=141.41808, "fx"=353.75125, "fy"=353.75125, "model"=4}, {"ID"=1, "Profile"=389858568, "fps"=6, "RS Stream"=3, "RS Format"=0, "index"=0, "width"=480, "height"=270, "ppx"=236.64972, "ppy"=141.41808, "fx"=353.75125, "fy"=353.75125, "model"=4}, {"ID"=1, "Profile"=389859848, "fps"=6, "RS Stream"=3, "RS Format"=0, "index"=0, "width"=480, "height"=270, "ppx"=236.64972, "ppy"=141.41808, "fx"=353.75125, "fy"=353.75125, "model"=4}, {"ID"=1, "Profile"=389867272, "fps"=6, "RS Stream"=3, "RS Format"=0, "index"=0, "width"=480, "height"=270, "ppx"=236.64972, "ppy"=141.41808, "fx"=353.75125, "fy"=353.75125, "model"=4}, {"ID"=1, "Profile"=389447736, "fps"=90, "RS Stream"=3, "RS Format"=0, "index"=0, "width"=424, "height"=240, "ppx"=209.02197, "ppy"=125.70496, "fx"=314.44556, "fy"=314.44556, "model"=4}, {"ID"=1, "Profile"=389447480, "fps"=90, "RS Stream"=3, "RS Format"=0, "index"=0, "width"=424, "height"=240, "ppx"=0.0, "ppy"=0.0, "fx"=0.0, "fy"=0.0, "model"=0}, {"ID"=2, "Profile"=389904168, "fps"=90, "RS Stream"=3, "RS Format"=0, "index"=2, "width"=424, "height"=240, "ppx"=209.02197, "ppy"=125.70496, "fx"=314.44556, "fy"=314.44556, "model"=4}, {"ID"=1, "Profile"=389450296, "fps"=90, "RS Stream"=3, "RS Format"=0, "index"=1, "width"=424, "height"=240, "ppx"=209.02197, "ppy"=125.70496, "fx"=314.44556, "fy"=314.44556, "model"=4}, {"ID"=1, "Profile"=389856520, "fps"=90, "RS Stream"=3, "RS Format"=0, "index"=0, "width"=424, "height"=240, "ppx"=209.02197, "ppy"=125.70496, "fx"=314.44556, "fy"=314.44556, "model"=4}, {"ID"=1, "Profile"=389447992, "fps"=90, "RS Stream"=3, "RS Format"=0, "index"=0, "width"=424, "height"=240, "ppx"=209.02197, "ppy"=125.70496, "fx"=314.44556, "fy"=314.44556, "model"=4}, {"ID"=1, "Profile"=119367816, "fps"=90, "RS Stream"=3, "RS Format"=0, "index"=0, "width"=424, "height"=240, "ppx"=209.02197, "ppy"=125.70496, "fx"=314.44556, "fy"=314.44556, "model"=4}, {"ID"=1, "Profile"=389447224, "fps"=90, "RS Stream"=3, "RS Format"=0, "index"=0, "width"=424, "height"=240, "ppx"=209.02197, "ppy"=125.70496, "fx"=314.44556, "fy"=314.44556, "model"=4}, {"ID"=1, "Profile"=389865736, "fps"=60, "RS Stream"=3, "RS Format"=0, "index"=0, "width"=424, "height"=240, "ppx"=209.02197, "ppy"=125.70496, "fx"=314.44556, "fy"=314.44556, "model"=4}, {"ID"=1, "Profile"=389870088, "fps"=60, "RS Stream"=3, "RS Format"=0, "index"=0, "width"=424, "height"=240, "ppx"=0.0, "ppy"=0.0, "fx"=0.0, "fy"=0.0, "model"=0}, {"ID"=2, "Profile"=389895464, "fps"=60, "RS Stream"=3, "RS Format"=0, "index"=2, "width"=424, "height"=240, "ppx"=209.02197, "ppy"=125.70496, "fx"=314.44556, "fy"=314.44556, "model"=4}, {"ID"=1, "Profile"=389454904, "fps"=60, "RS Stream"=3, "RS Format"=0, "index"=1, "width"=424, "height"=240, "ppx"=209.02197, "ppy"=125.70496, "fx"=314.44556, "fy"=314.44556, "model"=4}, {"ID"=1, "Profile"=389868552, "fps"=60, "RS Stream"=3, "RS Format"=0, "index"=0, "width"=424, "height"=240, "ppx"=209.02197, "ppy"=125.70496, "fx"=314.44556, "fy"=314.44556, "model"=4}, {"ID"=1, "Profile"=389869320, "fps"=60, "RS Stream"=3, "RS Format"=0, "index"=0, "width"=424, "height"=240, "ppx"=209.02197, "ppy"=125.70496, "fx"=314.44556, "fy"=314.44556, "model"=4}, {"ID"=1, "Profile"=389861384, "fps"=60, "RS Stream"=3, "RS Format"=0, "index"=0, "width"=424, "height"=240, "ppx"=209.02197, "ppy"=125.70496, "fx"=314.44556, "fy"=314.44556, "model"=4}, {"ID"=1, "Profile"=389866504, "fps"=60, "RS Stream"=3, "RS Format"=0, "index"=0, "width"=424, "height"=240, "ppx"=209.02197, "ppy"=125.70496, "fx"=314.44556, "fy"=314.44556, "model"=4}, {"ID"=1, "Profile"=389871880, "fps"=30, "RS Stream"=3, "RS Format"=0, "index"=0, "width"=424, "height"=240, "ppx"=209.02197, "ppy"=125.70496, "fx"=314.44556, "fy"=314.44556, "model"=4}, {"ID"=1, "Profile"=389869576, "fps"=30, "RS Stream"=3, "RS Format"=0, "index"=0, "width"=424, "height"=240, "ppx"=0.0, "ppy"=0.0, "fx"=0.0, "fy"=0.0, "model"=0}, {"ID"=2, "Profile"=389892648, "fps"=30, "RS Stream"=3, "RS Format"=0, "index"=2, "width"=424, "height"=240, "ppx"=209.02197, "ppy"=125.70496, "fx"=314.44556, "fy"=314.44556, "model"=4}, {"ID"=1, "Profile"=389460792, "fps"=30, "RS Stream"=3, "RS Format"=0, "index"=1, "width"=424, "height"=240, "ppx"=209.02197, "ppy"=125.70496, "fx"=314.44556, "fy"=314.44556, "model"=4}, {"ID"=1, "Profile"=389869064, "fps"=30, "RS Stream"=3, "RS Format"=0, "index"=0, "width"=424, "height"=240, "ppx"=209.02197, "ppy"=125.70496, "fx"=314.44556, "fy"=314.44556, "model"=4}, {"ID"=1, "Profile"=389869832, "fps"=30, "RS Stream"=3, "RS Format"=0, "index"=0, "width"=424, "height"=240, "ppx"=209.02197, "ppy"=125.70496, "fx"=314.44556, "fy"=314.44556, "model"=4}, {"ID"=1, "Profile"=389858824, "fps"=30, "RS Stream"=3, "RS Format"=0, "index"=0, "width"=424, "height"=240, "ppx"=209.02197, "ppy"=125.70496, "fx"=314.44556, "fy"=314.44556, "model"=4}, {"ID"=1, "Profile"=389862152, "fps"=30, "RS Stream"=3, "RS Format"=0, "index"=0, "width"=424, "height"=240, "ppx"=209.02197, "ppy"=125.70496, "fx"=314.44556, "fy"=314.44556, "model"=4}, {"ID"=1, "Profile"=389862408, "fps"=15, "RS Stream"=3, "RS Format"=0, "index"=0, "width"=424, "height"=240, "ppx"=209.02197, "ppy"=125.70496, "fx"=314.44556, "fy"=314.44556, "model"=4}, {"ID"=1, "Profile"=389871368, "fps"=15, "RS Stream"=3, "RS Format"=0, "index"=0, "width"=424, "height"=240, "ppx"=0.0, "ppy"=0.0, "fx"=0.0, "fy"=0.0, "model"=0}, {"ID"=2, "Profile"=389904424, "fps"=15, "RS Stream"=3, "RS Format"=0, "index"=2, "width"=424, "height"=240, "ppx"=209.02197, "ppy"=125.70496, "fx"=314.44556, "fy"=314.44556, "model"=4}, {"ID"=1, "Profile"=389457720, "fps"=15, "RS Stream"=3, "RS Format"=0, "index"=1, "width"=424, "height"=240, "ppx"=209.02197, "ppy"=125.70496, "fx"=314.44556, "fy"=314.44556, "model"=4}, {"ID"=1, "Profile"=389866248, "fps"=15, "RS Stream"=3, "RS Format"=0, "index"=0, "width"=424, "height"=240, "ppx"=209.02197, "ppy"=125.70496, "fx"=314.44556, "fy"=314.44556, "model"=4}, {"ID"=1, "Profile"=389864712, "fps"=15, "RS Stream"=3, "RS Format"=0, "index"=0, "width"=424, "height"=240, "ppx"=209.02197, "ppy"=125.70496, "fx"=314.44556, "fy"=314.44556, "model"=4}, {"ID"=1, "Profile"=389867016, "fps"=15, "RS Stream"=3, "RS Format"=0, "index"=0, "width"=424, "height"=240, "ppx"=209.02197, "ppy"=125.70496, "fx"=314.44556, "fy"=314.44556, "model"=4}, {"ID"=1, "Profile"=389864968, "fps"=15, "RS Stream"=3, "RS Format"=0, "index"=0, "width"=424, "height"=240, "ppx"=209.02197, "ppy"=125.70496, "fx"=314.44556, "fy"=314.44556, "model"=4}, {"ID"=1, "Profile"=389861640, "fps"=6, "RS Stream"=3, "RS Format"=0, "index"=0, "width"=424, "height"=240, "ppx"=209.02197, "ppy"=125.70496, "fx"=314.44556, "fy"=314.44556, "model"=4}, {"ID"=1, "Profile"=389859080, "fps"=6, "RS Stream"=3, "RS Format"=0, "index"=0, "width"=424, "height"=240, "ppx"=0.0, "ppy"=0.0, "fx"=0.0, "fy"=0.0, "model"=0}, {"ID"=2, "Profile"=389898792, "fps"=6, "RS Stream"=3, "RS Format"=0, "index"=2, "width"=424, "height"=240, "ppx"=209.02197, "ppy"=125.70496, "fx"=314.44556, "fy"=314.44556, "model"=4}, {"ID"=1, "Profile"=389457976, "fps"=6, "RS Stream"=3, "RS Format"=0, "index"=1, "width"=424, "height"=240, "ppx"=209.02197, "ppy"=125.70496, "fx"=314.44556, "fy"=314.44556, "model"=4}, {"ID"=1, "Profile"=389868808, "fps"=6, "RS Stream"=3, "RS Format"=0, "index"=0, "width"=424, "height"=240, "ppx"=209.02197, "ppy"=125.70496, "fx"=314.44556, "fy"=314.44556, "model"=4}, {"ID"=1, "Profile"=389868296, "fps"=6, "RS Stream"=3, "RS Format"=0, "index"=0, "width"=424, "height"=240, "ppx"=209.02197, "ppy"=125.70496, "fx"=314.44556, "fy"=314.44556, "model"=4}, {"ID"=1, "Profile"=389857288, "fps"=6, "RS Stream"=3, "RS Format"=0, "index"=0, "width"=424, "height"=240, "ppx"=209.02197, "ppy"=125.70496, "fx"=314.44556, "fy"=314.44556, "model"=4}, {"ID"=1, "Profile"=389871624, "fps"=6, "RS Stream"=3, "RS Format"=0, "index"=0, "width"=424, "height"=240, "ppx"=209.02197, "ppy"=125.70496, "fx"=314.44556, "fy"=314.44556, "model"=4}, {"ID"=0, "Profile"=389455416, "fps"=30, "RS Stream"=1, "RS Format"=0, "index"=0, "width"=1280, "height"=720, "ppx"=631.0659, "ppy"=377.11487, "fx"=943.3367, "fy"=943.3367, "model"=4}, {"ID"=0, "Profile"=389446456, "fps"=30, "RS Stream"=1, "RS Format"=0, "index"=0, "width"=1280, "height"=720, "ppx"=631.0659, "ppy"=377.11487, "fx"=943.3367, "fy"=943.3367, "model"=4}, {"ID"=0, "Profile"=389455672, "fps"=30, "RS Stream"=1, "RS Format"=0, "index"=0, "width"=640, "height"=480, "ppx"=314.04395, "ppy"=251.40993, "fx"=628.8911, "fy"=628.8911, "model"=4}, {"ID"=0, "Profile"=389450552, "fps"=30, "RS Stream"=1, "RS Format"=0, "index"=0, "width"=640, "height"=480, "ppx"=314.04395, "ppy"=251.40993, "fx"=628.8911, "fy"=628.8911, "model"=4}] {"model" items=["RS_DISTORTION_NONE", "RS_DISTORTION_MODIFIED_BROWN_CONRADY", "RS_DISTORTION_INVERSE_BROWN_CONRADY", "RS_DISTORTION_FTHETA", "RS_DISTORTION_BROWN_CONRADY", "RS_DISTORTION_COUNT"]; "RS Stream" items=["    RS2_STREAM_ANY,", "    RS2_STREAM_DEPTH                            , /**< Native stream of depth data produced by RealSense device */", "    RS2_STREAM_COLOR                            , /**< Native stream of color data captured by RealSense device */", "    RS2_STREAM_INFRARED                         , /**< Native stream of infrared data captured by RealSense device */", "    RS2_STREAM_FISHEYE                          , /**< Native stream of fish-eye (wide) data captured from the dedicate motion camera */", "    RS2_STREAM_GYRO                             , /**< Native stream of gyroscope motion data produced by RealSense device */", "    RS2_STREAM_ACCEL                            , /**< Native stream of accelerometer motion data produced by RealSense device */", "    RS2_STREAM_GPIO                             , /**< Signals from external device connected through GPIO */", "    RS2_STREAM_POSE                             , /**< 6 Degrees of Freedom pose data, calculated by RealSense device */", "    RS2_STREAM_CONFIDENCE,", "    RS2_STREAM_COUNT"]}, 11 "Stream selection":T3(ring)=enum."Rectified L + R") -> (0 "error out":errorcluster, 2 "number of resolutions":i32, 3 "Available Stream Pairs":T1)   [LabVIEW 2017, in "libRealSense3.lvlib"]
doc: "This VI looks at all the available streams and sorts them into the prescribed pairs for easier handling."
uses:
  libRealSense3.lvlib
panel:
  # "RS3 Decode Stream Pairs"
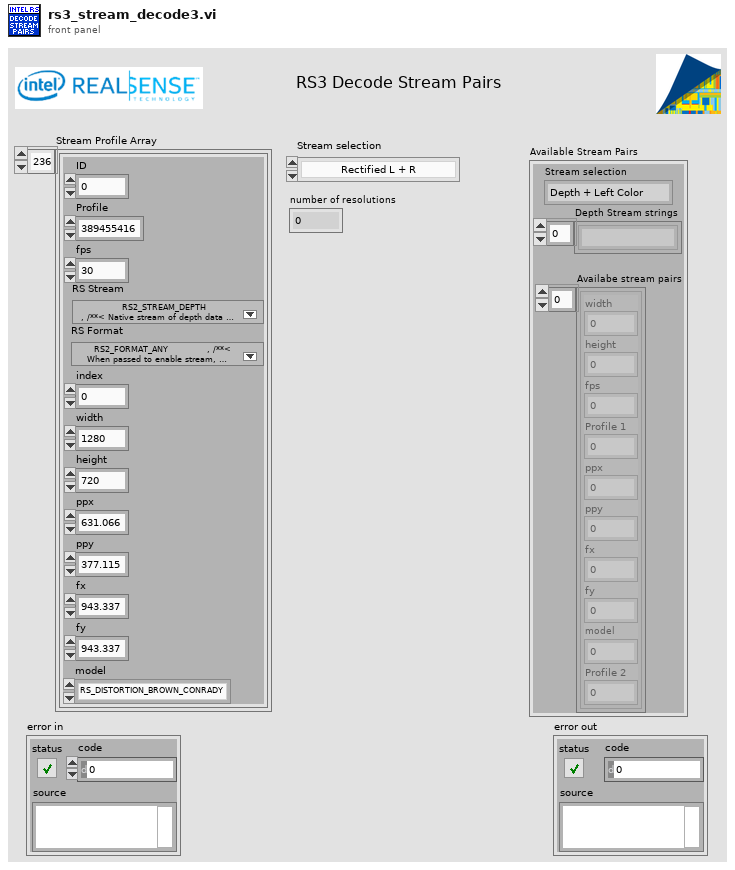
[diagram p1: front panel]
types:
  T1 = cluster{"Stream selection":enum16{"Depth + Left Color", "Unrectified L + R", "Rectified L + R", "Depth Only", "RGB ext. Only", "Depth + L Monochrome"}, "Depth Stream strings":string[], "Availabe stream pairs":cluster{"width":i32, "height":i32, "fps":i32, "Profile 1":u64, "ppx":sgl, "ppy":sgl, "fx":sgl, "fy":sgl, "model":u32, "Profile 2":u64}[]}
  T2 = cluster{"ID":i32, "Profile":u64, "fps":i32, "RS Stream":u16, "RS Format":u16, "index":u16, "width":u16, "height":u16, "ppx":sgl, "ppy":sgl, "fx":sgl, "fy":sgl, "model":u32}[]
  T3 = enum16{"Depth + Left Color", "Unrectified L + R", "Rectified L + R", "Depth Only", "RGB ext. Only", "Depth + L Monochrome", "Depth Only(compressed)"}
  T4 = cluster{"width":i32, "height":i32, "fps":i32, "Profile":u64, "ppx":sgl, "ppy":sgl, "fx":sgl, "fy":sgl, "model":u32}[]
  T5 = cluster{"Stream selection":enum16{"Depth + Left Color", "Unrectified L + R", "Rectified L + R", "Depth Only", "RGB ext. Only", "Depth + L Monochrome"}, "Depth Stream strings":string[], cluster{"width":i32, "height":i32, "fps":i32, "Profile 1":u64, "ppx":sgl, "ppy":sgl, "fx":sgl, "fy":sgl, "model":u32, "Profile 2":u64}[]}
  T6 = cluster{"width":i32, "height":i32, "fps":i32, "Profile 1":u64, "ppx":sgl, "ppy":sgl, "fx":sgl, "fy":sgl, "model":u32, "Profile 2":u64}
  T7 = cluster{"width":i32, "height":i32, "fps":i32, "Profile":u64, "ppx":sgl, "ppy":sgl, "fx":sgl, "fy":sgl, "model":u32, "Profile":u64}
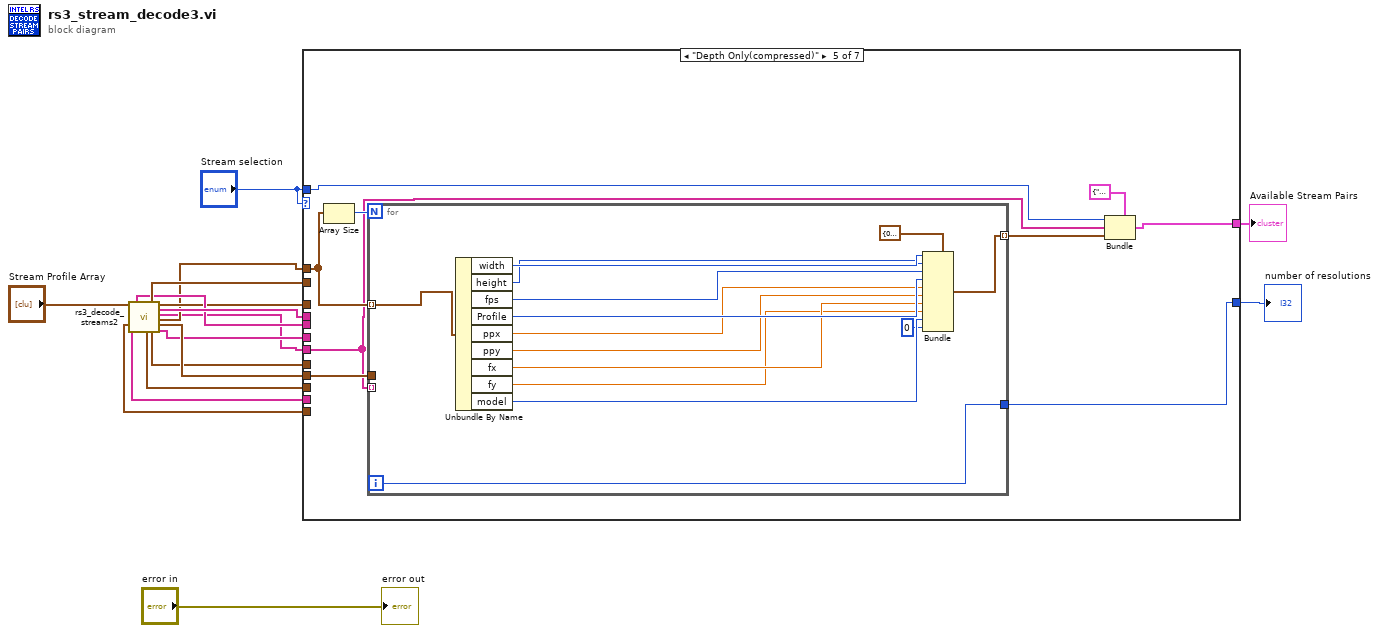
[diagram p0: block diagram]
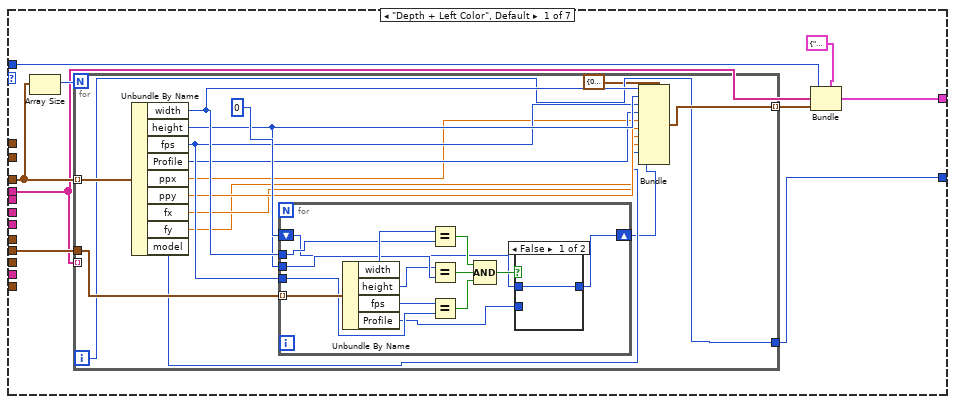
[diagram p2: hidden frame]
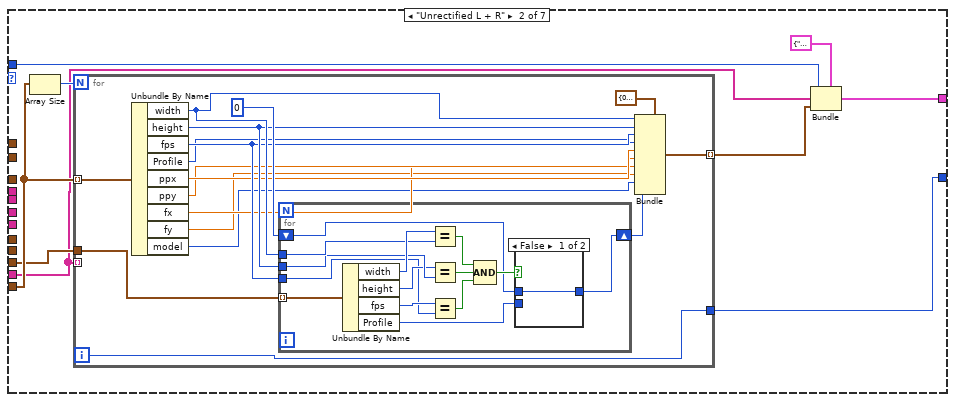
[diagram p4: hidden frame]
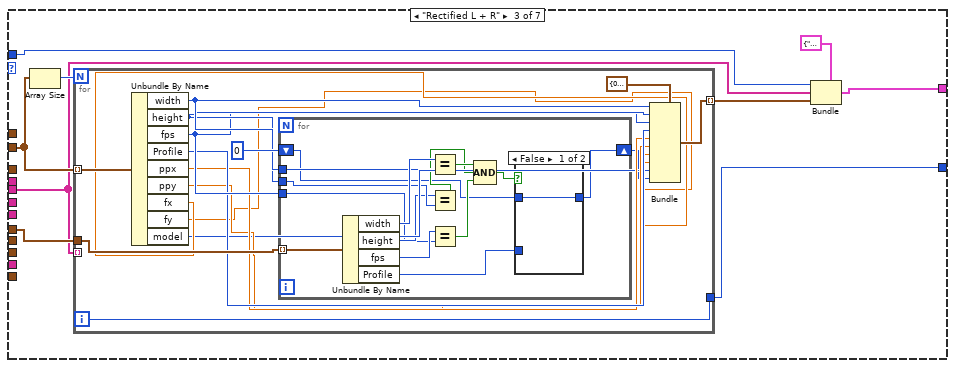
[diagram p6: hidden frame]
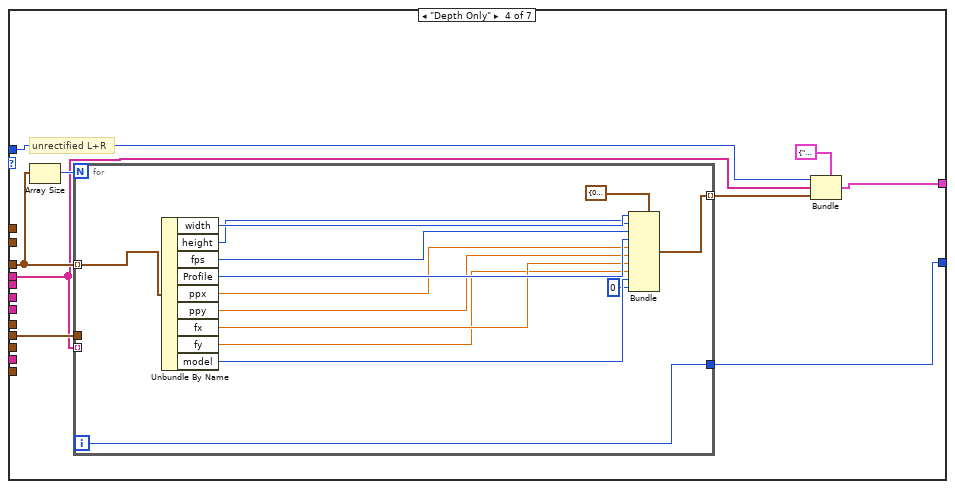
[diagram p8: hidden frame]
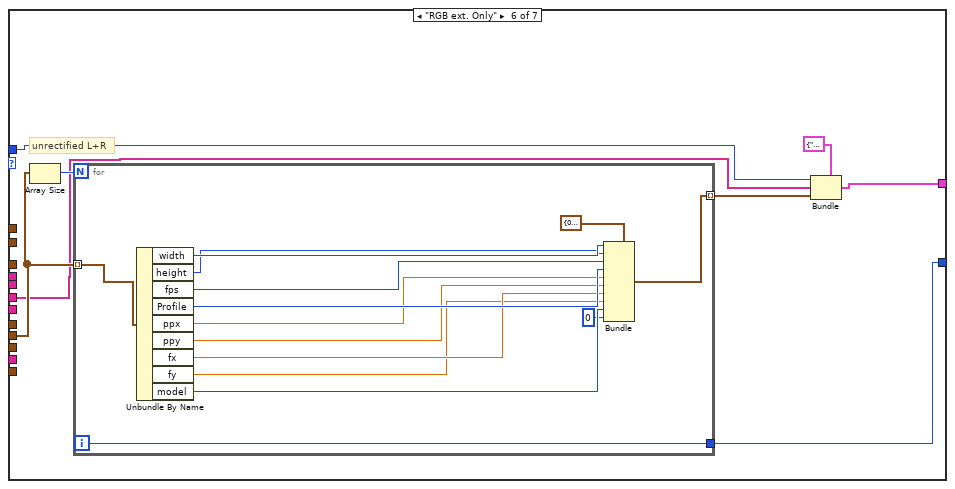
[diagram p9: hidden frame]
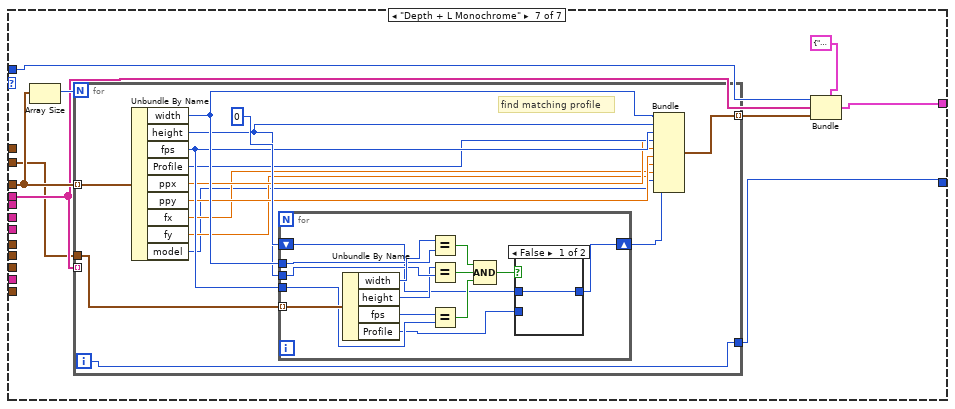
[diagram p10: hidden frame]
diagram:
  n1 = call "rs3_decode_streams2.vi"("Stream profile array"="Stream Profile Array") -> (4:"Unrectified L IR"=w13:T4, 5:"Unrectified L IR"=w14:string[], "IR Left Array"=w8:string[], "Unrectified R  IR"=w12:T4, "IR left"=w10:T4, "IR Right"=w9:T4, "Depth Stream"=w3:T4, "Depth Stream strings"=w15:string[], "Depth Stream strings Compress"=w1:string[], "Depth Stream Compress."=w2:T4, "Color Left"=w17:T4, "Color Left Array"=w7:string[])  [unwired: 3 in, 4 out]
  n2 = case shown="\"Depth Only(compressed)\"" "Stream selection" {
    tunnel: w17 -> [w26 _ _ w149 w172 w191 _]
    tunnel: w3 -> [w25 _ _ w148 _ _ w217]
    tunnel: w15 -> [w22 _ _ w145 _ _ w213]
    tunnel: w14 -> [_ w63 _ _ _ _ _]
    tunnel: w13 -> [_ w65 _ _ _ _ _]
    tunnel: w12 -> [_ w64 _ _ _ _ _]
    tunnel: "Stream selection" -> [w23 w66 w107 w146 w170 w193 w215]
    tunnel: [w19 w61 w100 w143 w168 w189 w214] -> w5
    tunnel: w10 -> [_ _ w105 _ _ _ w212]
    tunnel: w9 -> [_ _ w104 _ _ _ _]
    tunnel: w8 -> [_ _ w103 _ _ _ _]
    tunnel: w7 -> [_ _ _ _ _ w190 _]
    tunnel: [w18 w59 w101 w141 w166 w187 w209] -> w4
    tunnel: w2 -> [_ _ _ _ w165 _ _]
    tunnel: w1 -> [_ _ _ _ w164 _ _]
    frame "Depth + Left Color", Default {
      n3 = Array Size(array=w25) -> (size(s)=w24:i32)
      n4 = for {
        N: w24 -> [_]
        tunnel: w25 -> [w40] mode=indexing
        tunnel: w26 -> [w42]
        tunnel: w22 -> [_] mode=indexing
        tunnel: [w29] -> w21 mode=indexing
        tunnel: [w28] -> w18
        i -> [w28]
        n5 = Unbundle By Name(w40) -> ("width"=w39:i32, "height"=w38:i32, "fps"=w37:i32, "Profile"=w36:u64, "ppx"=w35:sgl, "ppy"=w34:sgl, "fx"=w33:sgl, "fy"=w32:sgl, "model"=w31:u32)
        n6 = for {
          tunnel: w42 -> [w56] mode=indexing
          tunnel: w39 -> [w54]
          tunnel: w38 -> [w53]
          tunnel: w37 -> [w50]
          shift-right: [w45] -> w30
          shift-left: u64 0 ("Profile") -> [w43]
          n7 = Unbundle By Name(w56) -> ("width"=w55:i32, "height"=w52:i32, "fps"=w51:i32, "Profile"=w44:u64)
          n8 = Equal?(x=w55, y=w54) -> (x = y?=w49:bool)
          n9 = Equal?(x=w52, y=w53) -> (x = y?=w48:bool)
          n10 = Equal?(x=w51, y=w50) -> (x = y?=w47:bool)
          n11 = Compound Arithmetic op=AND(w49, w48, w47) -> (w46:bool)
          n12 = case shown="False" w46 {
            tunnel: [w57 w58] -> w45
            tunnel: w44 -> [_ w58]
            tunnel: w43 -> [w57 _]
            frame False {
            }
            frame True {
            }
          }
        }
        n13 = Bundle(cluster=T6 {"width"=0, "height"=0, "fps"=0, "Profile 1"=0, "ppx"=0.0, "ppy"=0.0, "fx"=0.0, "fy"=0.0, "model"=4, "Profile 2"=0} ("Selected stream"), "width"=w39, "height"=w38, "fps"=w37, "Profile 1"=w36, "ppx"=w35, "ppy"=w34, "fx"=w33, "fy"=w32, "model"=w31, "Profile 2"=w30) -> (w29:T6)
      }
      n14 = Bundle(cluster=T5 {"Stream selection"=enum."Depth + Left Color", "Depth Stream strings"=[], []} ("output cluster"), "Stream selection"=w23, "Depth Stream strings"=w22, w21) -> (w19:T5)
    }
    frame "Unrectified L + R" {
      n15 = Array Size(array=w65) -> (size(s)=w67:i32)
      n16 = for {
        N: w67 -> [_]
        tunnel: w65 -> [w81] mode=indexing
        tunnel: w64 -> [w83]
        tunnel: w63 -> [_] mode=indexing
        tunnel: [w69] -> w62 mode=indexing
        tunnel: [w68] -> w59
        i -> [w68]
        n17 = Unbundle By Name(w81) -> ("width"=w79:i32, "height"=w78:i32, "fps"=w77:i32, "Profile"=w76:u64, "ppx"=w75:sgl, "ppy"=w74:sgl, "fx"=w73:sgl, "fy"=w72:sgl, "model"=w71:u32)
        n18 = for {
          tunnel: w83 -> [w97] mode=indexing
          tunnel: w79 -> [w95]
          tunnel: w78 -> [w94]
          tunnel: w77 -> [w91]
          shift-right: [w86] -> w70
          shift-left: u64 0 ("Profile") -> [w84]
          n19 = Unbundle By Name(w97) -> ("width"=w96:i32, "height"=w93:i32, "fps"=w92:i32, "Profile"=w85:u64)
          n20 = Equal?(x=w96, y=w95) -> (x = y?=w90:bool)
          n21 = Equal?(x=w93, y=w94) -> (x = y?=w89:bool)
          n22 = Equal?(x=w92, y=w91) -> (x = y?=w88:bool)
          n23 = Compound Arithmetic op=AND(w90, w89, w88) -> (w87:bool)
          n24 = case shown="False" w87 {
            tunnel: [w98 w99] -> w86
            tunnel: w85 -> [_ w99]
            tunnel: w84 -> [w98 _]
            frame False {
            }
            frame True {
            }
          }
        }
        n25 = Bundle(cluster=T6 {"width"=0, "height"=0, "fps"=0, "Profile 1"=0, "ppx"=0.0, "ppy"=0.0, "fx"=0.0, "fy"=0.0, "model"=4, "Profile 2"=0} ("Selected stream"), "width"=w79, "height"=w78, "fps"=w77, "Profile 1"=w76, "ppx"=w75, "ppy"=w74, "fx"=w73, "fy"=w72, "model"=w71, "Profile 2"=w70) -> (w69:T6)
      }
      n26 = Bundle(cluster=T5 {"Stream selection"=enum."Depth + Left Color", "Depth Stream strings"=[], []} ("output cluster"), "Stream selection"=w66, "Depth Stream strings"=w63, w62) -> (w61:T5)
    }
    frame "Rectified L + R" {
      n27 = Array Size(array=w105) -> (size(s)=w108:i32)
      n28 = for {
        N: w108 -> [_]
        tunnel: w105 -> [w122] mode=indexing
        tunnel: w104 -> [w124]
        tunnel: w103 -> [_] mode=indexing
        tunnel: [w120] -> w106 mode=indexing
        tunnel: [w109] -> w101
        i -> [w109]
        n29 = Unbundle By Name(w122) -> ("width"=w119:i32, "height"=w118:i32, "fps"=w117:i32, "Profile"=w116:u64, "ppx"=w115:sgl, "ppy"=w114:sgl, "fx"=w113:sgl, "fy"=w112:sgl, "model"=w111:u32)
        n30 = for {
          tunnel: w124 -> [w138] mode=indexing
          tunnel: w119 -> [w136]
          tunnel: w118 -> [w135]
          tunnel: w117 -> [w132]
          shift-right: [w127] -> w110
          shift-left: u64 0 ("Profile") -> [w125]
          n31 = Unbundle By Name(w138) -> ("width"=w137:i32, "height"=w134:i32, "fps"=w133:i32, "Profile"=w126:u64)
          n32 = Equal?(x=w137, y=w136) -> (x = y?=w131:bool)
          n33 = Equal?(x=w134, y=w135) -> (x = y?=w130:bool)
          n34 = Equal?(x=w133, y=w132) -> (x = y?=w129:bool)
          n35 = Compound Arithmetic op=AND(w131, w130, w129) -> (w128:bool)
          n36 = case shown="False" w128 {
            tunnel: [w139 w140] -> w127
            tunnel: w126 -> [_ w140]
            tunnel: w125 -> [w139 _]
            frame False {
            }
            frame True {
            }
          }
        }
        n37 = Bundle(cluster=T6 {"width"=0, "height"=0, "fps"=0, "Profile 1"=0, "ppx"=0.0, "ppy"=0.0, "fx"=0.0, "fy"=0.0, "model"=4, "Profile 2"=0} ("Selected stream"), "width"=w119, "height"=w118, "fps"=w117, "Profile 1"=w116, "ppx"=w115, "ppy"=w114, "fx"=w113, "fy"=w112, "model"=w111, "Profile 2"=w110) -> (w120:T6)
      }
      n38 = Bundle(cluster=T5 {"Stream selection"=enum."Depth + Left Color", "Depth Stream strings"=[], []} ("output cluster"), "Stream selection"=w107, "Depth Stream strings"=w103, w106) -> (w100:T5)
    }
    frame "Depth Only" {
      # "unrectified L+R"
      n39 = Array Size(array=w148) -> (size(s)=w147:i32)
      n40 = for {
        N: w147 -> [_]
        tunnel: w148 -> [w162] mode=indexing
        tunnel: w149 -> [_]
        tunnel: w145 -> [_] mode=indexing
        tunnel: [w151] -> w144 mode=indexing
        tunnel: [w150] -> w141
        i -> [w150]
        n41 = Unbundle By Name(w162) -> ("width"=w161:i32, "height"=w160:i32, "fps"=w159:i32, "Profile"=w158:u64, "ppx"=w157:sgl, "ppy"=w156:sgl, "fx"=w155:sgl, "fy"=w154:sgl, "model"=w153:u32)
        n42 = Bundle(cluster=T6 {"width"=0, "height"=0, "fps"=0, "Profile 1"=0, "ppx"=0.0, "ppy"=0.0, "fx"=0.0, "fy"=0.0, "model"=4, "Profile 2"=0} ("Selected stream"), "width"=w161, "height"=w160, "fps"=w159, "Profile 1"=w158, "ppx"=w157, "ppy"=w156, "fx"=w155, "fy"=w154, "model"=w153, "Profile 2"=u64 0) -> (w151:T6)
      }
      n43 = Bundle(cluster=T5 {"Stream selection"=enum."Depth + Left Color", "Depth Stream strings"=[], []} ("output cluster"), "Stream selection"=w146, "Depth Stream strings"=w145, w144) -> (w143:T5)
    }
    frame "Depth Only(compressed)" {
      n44 = Array Size(array=w165) -> (size(s)=w171:i32)
      n45 = for {
        N: w171 -> [_]
        tunnel: w165 -> [w185] mode=indexing
        tunnel: w172 -> [_]
        tunnel: w164 -> [_] mode=indexing
        tunnel: [w174] -> w169 mode=indexing
        tunnel: [w173] -> w166
        i -> [w173]
        n46 = Unbundle By Name(w185) -> ("width"=w184:i32, "height"=w183:i32, "fps"=w182:i32, "Profile"=w181:u64, "ppx"=w180:sgl, "ppy"=w179:sgl, "fx"=w178:sgl, "fy"=w177:sgl, "model"=w176:u32)
        n47 = Bundle(cluster=T6 {"width"=0, "height"=0, "fps"=0, "Profile 1"=0, "ppx"=0.0, "ppy"=0.0, "fx"=0.0, "fy"=0.0, "model"=4, "Profile 2"=0} ("Selected stream"), "width"=w184, "height"=w183, "fps"=w182, "Profile 1"=w181, "ppx"=w180, "ppy"=w179, "fx"=w178, "fy"=w177, "model"=w176, "Profile 2"=u64 0) -> (w174:T6)
      }
      n48 = Bundle(cluster=T5 {"Stream selection"=enum."Depth + Left Color", "Depth Stream strings"=[], []} ("output cluster"), "Stream selection"=w170, "Depth Stream strings"=w164, w169) -> (w168:T5)
    }
    frame "RGB ext. Only" {
      # "unrectified L+R"
      n49 = Array Size(array=w191) -> (size(s)=w194:i32)
      n50 = for {
        N: w194 -> [_]
        tunnel: w191 -> [w196] mode=indexing
        tunnel: [w197] -> w192 mode=indexing
        tunnel: [w195] -> w187
        i -> [w195]
        n51 = Unbundle By Name(w196) -> ("width"=w207:i32, "height"=w206:i32, "fps"=w205:i32, "Profile"=w204:u64, "ppx"=w203:sgl, "ppy"=w202:sgl, "fx"=w201:sgl, "fy"=w200:sgl, "model"=w199:u32)
        n52 = Bundle(cluster=T6 {"width"=0, "height"=0, "fps"=0, "Profile 1"=0, "ppx"=0.0, "ppy"=0.0, "fx"=0.0, "fy"=0.0, "model"=4, "Profile 2"=0} ("Selected stream"), "width"=w207, "height"=w206, "fps"=w205, "Profile 1"=w204, "ppx"=w203, "ppy"=w202, "fx"=w201, "fy"=w200, "model"=w199, "Profile 2"=u64 0) -> (w197:T6)
      }
      n53 = Bundle(cluster=T5 {"Stream selection"=enum."Depth + Left Color", "Depth Stream strings"=[], []} ("output cluster"), "Stream selection"=w193, "Depth Stream strings"=w190, w192) -> (w189:T5)
    }
    frame "Depth + L Monochrome" {
      n54 = Array Size(array=w217) -> (size(s)=w216:i32)
      n55 = for {
        N: w216 -> [_]
        tunnel: w217 -> [w230] mode=indexing
        tunnel: w212 -> [w232]
        tunnel: w213 -> [_] mode=indexing
        tunnel: [w219] -> w211 mode=indexing
        tunnel: [w218] -> w209
        i -> [w218]
        # "find matching profile"
        n56 = Unbundle By Name(w230) -> ("width"=w229:i32, "height"=w228:i32, "fps"=w227:i32, "Profile"=w226:u64, "ppx"=w225:sgl, "ppy"=w224:sgl, "fx"=w223:sgl, "fy"=w222:sgl, "model"=w221:u32)
        n57 = for {
          tunnel: w232 -> [w246] mode=indexing
          tunnel: w229 -> [w244]
          tunnel: w228 -> [w243]
          tunnel: w227 -> [w240]
          shift-right: [w235] -> w220
          shift-left: u64 0 ("Profile") -> [w233]
          n58 = Unbundle By Name(w246) -> ("width"=w245:i32, "height"=w242:i32, "fps"=w241:i32, "Profile"=w234:u64)
          n59 = Equal?(x=w245, y=w244) -> (x = y?=w239:bool)
          n60 = Equal?(x=w242, y=w243) -> (x = y?=w238:bool)
          n61 = Equal?(x=w241, y=w240) -> (x = y?=w237:bool)
          n62 = Compound Arithmetic op=AND(w239, w238, w237) -> (w236:bool)
          n63 = case shown="False" w236 {
            tunnel: [w247 w248] -> w235
            tunnel: w234 -> [_ w248]
            tunnel: w233 -> [w247 _]
            frame False {
            }
            frame True {
            }
          }
        }
        n64 = Bundle("width"=w229, "height"=w228, "fps"=w227, "Profile"=w226, "ppx"=w225, "ppy"=w224, "fx"=w223, "fy"=w222, "model"=w221, "Profile"=w220) -> (w219:T7)  [unwired: 1 in]
      }
      n65 = Bundle(cluster=T5 {"Stream selection"=enum."Depth + Left Color", "Depth Stream strings"=[], []} ("output cluster"), "Stream selection"=w215, "Depth Stream strings"=w213, w211) -> (w214:T5)
    }
  }
  "number of resolutions" <- w4
  "Available Stream Pairs" <- w5
  "error out" <- "error in"
